vi "_TopToCurrent.vi"(11 "Next States in":T2) -> (2 "Next States out":T2, 3 "Next State":T1)   [LabVIEW 2020]
uses:
  TDefs/States.ctl
  TDefs/State.ctl
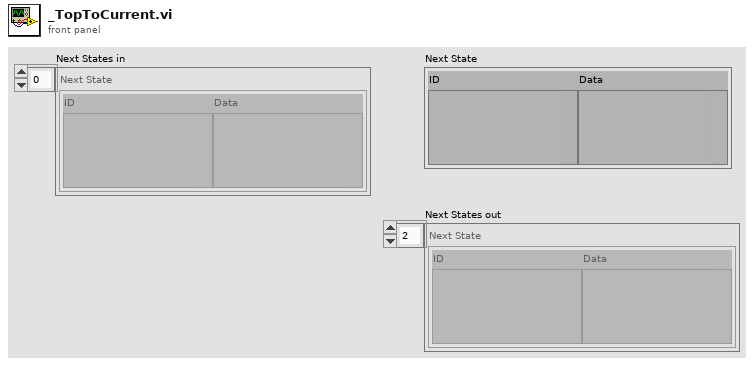
[diagram p1: front panel]
types:
  T1 = typedef "State.ctl" = cluster{"ID":variant, "Data":variant}
  T2 = typedef "States.ctl" = T1[]
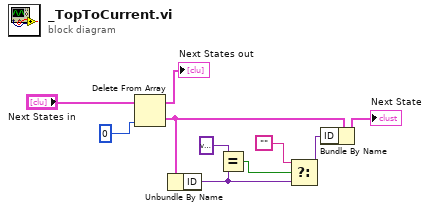
[diagram p0: block diagram]
diagram:
  n1 = Delete From Array(array="Next States in", index=0) -> (deleted portion=w7:T1, array with subset deleted=→"Next States out":T2)  [unwired: 1 in]
  n2 = Unbundle By Name(w7) -> ("ID"=w2:variant)
  n3 = Equal?(x=variant ("y"), y=w2) -> (x = y?=w4:bool)
  n4 = Select(t="", s=w4, f=w2) -> (s? t:f=w1:variant)
  n5 = Bundle By Name(cluster=w7, "ID"=w1) -> (→"Next State":T1)
